vi "Check if Windows Process Exists.vi"(8 "error in (no error)":errorcluster, 11 "str":string="softioc.exe") -> (0 "error out":errorcluster, 2 "process exist?":bool=TRUE, 3 "service name":string="NITaggerService", 4 "console out":string="SERVICE_NAME: NITaggerService\r\nTRUE")   [LabVIEW 2017]
doc: "Checks whether a Windows process matching str is running, by querying the task list through System Exec. Returns the matched process name and the raw console output."
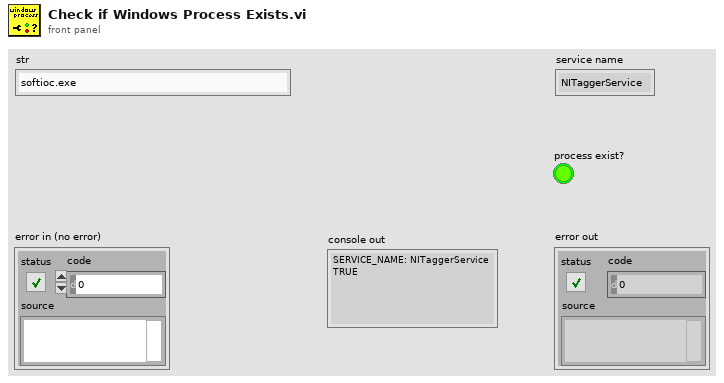
[diagram p1: front panel]
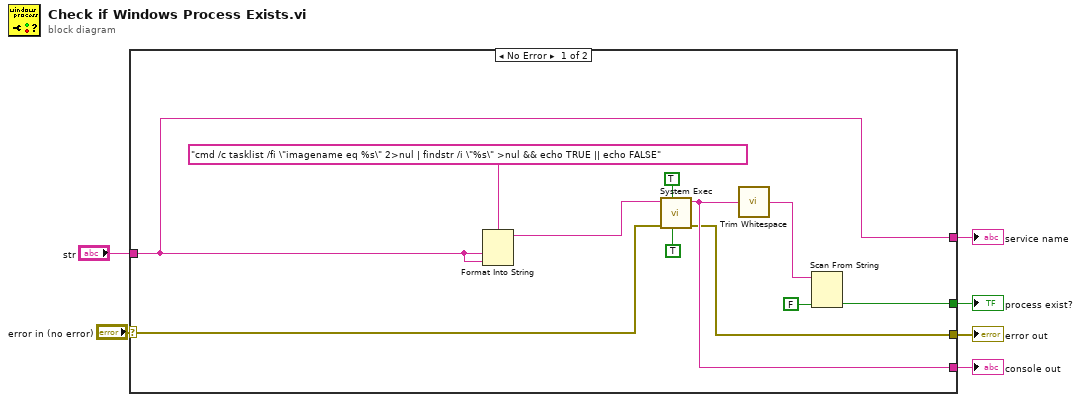
[diagram p0: block diagram]
diagram:
  n1 = case shown="No Error" "error in (no error)" {
    selector: "error in (no error)" -> [w11 w18]
    tunnel: [w8 _] -> w6
    tunnel: [w15 _] -> w5
    tunnel: "str" -> [w8 _]
    tunnel: [w12 _] -> w3
    tunnel: [w10 w18] -> w1
    frame No Error {
      n2 = Format Into String(format string="cmd /c tasklist /fi \"imagename eq %s\" 2>nul | findstr /i \"%s\" >nul && echo TRUE || echo FALSE" ("command line"), w8, w8) -> (resulting string=w13:string)  [unwired: 2 in, 1 out]
      n3 = call <vilib>:"System Exec.vi"("run minimized? (F)"=TRUE, "wait until completion? (T)"=TRUE, "error in (no error)"=w11, "command line"=w13) -> ("error out"=w10:errorcluster, "standard output"=w12:string)  [unwired: 4 in, 2 out]
      n4 = call <vilib>:"Trim Whitespace.vi"("string"=w12) -> ("trimmed string"=w9:string)  [unwired: 1 in]
      n5 = Scan From String(input string=w9, default 1=FALSE) -> (output 1=w15:bool)  [unwired: 3 in, 3 out]
    }
    frame Error {
    }
  }
  "console out" <- w3
  "service name" <- w6
  "process exist?" <- w5
  "error out" <- w1
